vi "Robot Main.vi"() -> ()   [LabVIEW 2011]
doc: "This VI imlements the framework and scheduler for your robotics program. It should not be necessary to modify the framework. You are expected to add your code to the VIs called from Robot Main, the ones located in the Team Code within the project."
uses:
  <vilib>/Rock Robotics/WPI/Camera/WPI_CameraImageSize.ctl
  Robot Global Data.vi
panel:
  out "Timings":cluster{"Call Name":string, "Delta (ms)":u32}[](array[cluster])
  in  "Image Size":T1=enum."320x240"
  in  "Enable Vision":bool
  in  "Finish":bool
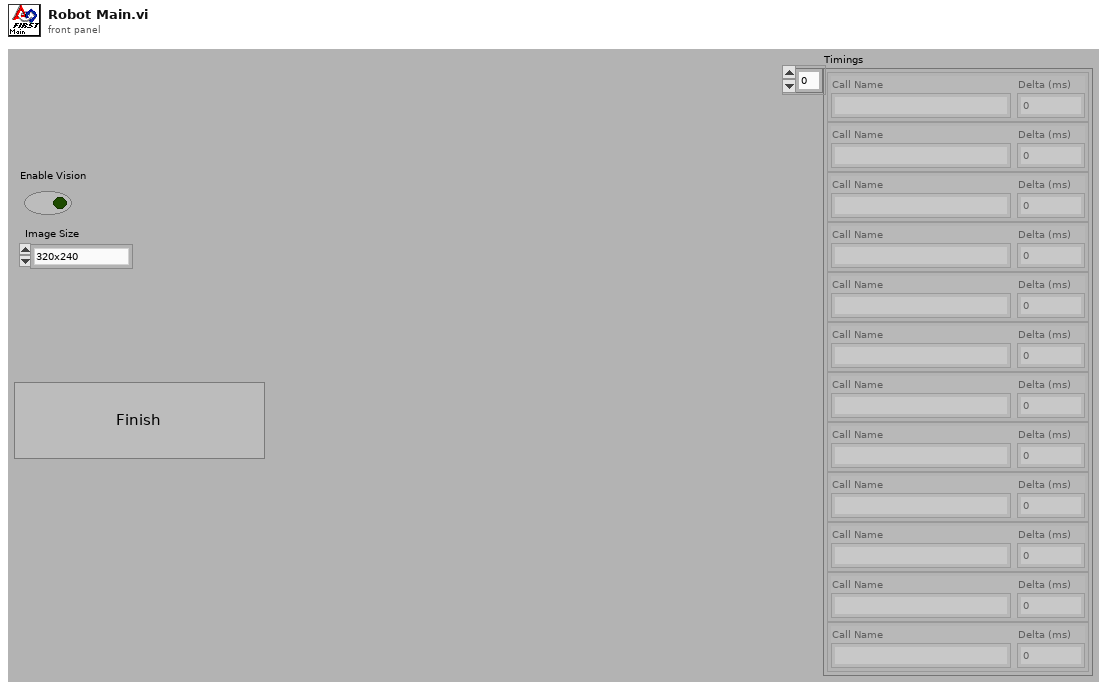
[diagram p1: front panel]
types:
  T1 = typedef "WPI_CameraImageSize.ctl" = enum16{"640x480", "320x240", "160x120"}
  T2 = typedef "WPI_DriverStationMatch Info.ctl" = cluster{"Autonomous Elapsed Seconds":dbl, "TeleOp Elapsed Seconds":dbl, "Disabled Elapsed Seconds":dbl, "Visited Autonomous":bool, "Visited TeleOp":bool, "Visited Disabled":bool, "Autonomous Settings":cluster{"Autonomous Style":enum16{"Iterative", "Independent"}, "VI Refnum":refnum<vi>}}
  T3 = typedef "WPI_DriverStationDerivedRobotMode.ctl" = enum16{"Init", "Execute", "Stop"}
  T4 = typedef "WPI_DriverStationRobotMode.ctl" = enum16{"Autonomous Disabled", "Autonomous Enabled", "Teleop Disabled", "Teleop Enabled", "Timeout", "Finish"}
  T5 = typedef "WPI_EncoderDevRef.ctl" = cluster{"DevStatus":errorcluster, "EncoderIndex":T6, "CounterIndex":T7, "DistancePerCount":dbl, "Decoding Type":T8}
  T6 = typedef "FPGA_EncoderIdx.ctl" = enum8{"Enc 0", "Enc 1", "Enc 2", "Enc 3", "Invalid"}
  T7 = typedef "FPGA_CounterCtrSystemIndex.ctl" = enum8{"Ctr 0", "Ctr 1", "Ctr 2", "Ctr 3", "Ctr 4", "Ctr 5", "Ctr 6", "Ctr 7", "Invalid"}
  T8 = typedef "WPI_EncoderType.ctl" = enum16{"1x", "2x", "4x"}
  T9 = typedef "WPI_GyroDevRef.ctl" = cluster{"DevStatus":errorcluster, "Analog Module":T10, "Analog Channel":T11, "Offset":dbl, "Gain (VoltsPerDegree/Second)":dbl}
  T10 = typedef "FPGA_TypedefAnalogModule.ctl" = enum16{"Analog Module 1", "Analog Module 2"}
  T11 = typedef "FPGA_AIChannel.ctl" = enum8{"AI 1", "AI 2", "AI 3", "AI 4", "AI 5", "AI 6", "AI 7", "AI 8", "Invalid"}
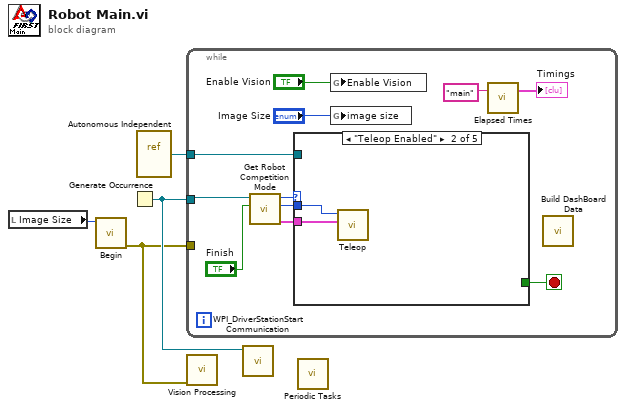
[diagram p0: block diagram]
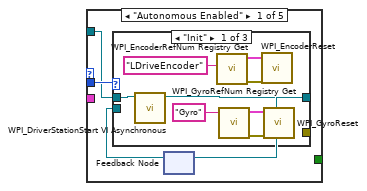
[diagram p2: hidden frame]
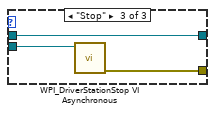
[diagram p4: hidden frame]
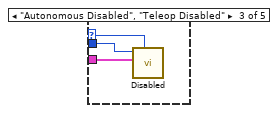
[diagram p5: hidden frame]
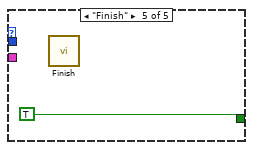
[diagram p7: hidden frame]
diagram:
  n1 = local read "Image Size"() -> (w3:T1)
  n2 = call "Begin.vi"("Image Size"=w3) -> ("error out"=w1:errorcluster)  [unwired: 10 out]
  n3 = Generate Occurrence() -> (w4:refnum<k4>)
  n4 = vi-ref "Autonomous Independent.vi"() -> (w2:refnum<vi>)
  n5 = while {
    tunnel: w4 -> [w13]
    tunnel: w1 -> [_]
    tunnel: w2 -> [w8]
    stop <- w10 stop-if-true
    n6 = call "Get Robot Competition Mode.vi"("Finish"="Finish", "DS Occurrence"=w13) -> ("Match Info out"=w11:T2, "Call Context"=w15:T3, "Robot Mode"=w14:T4)  [unwired: 7 out]
    n7 = case shown="\"Teleop Enabled\"" w14 {
      selector: w14 -> [_ _ w34 _ _]
      tunnel: w15 -> [w19 w33 w36 _ _]
      tunnel: w11 -> [_ w32 w35 _ _]
      tunnel: [_ _ _ _ TRUE] -> w10
      tunnel: w8 -> [w18 _ _ _ _]
      frame "Autonomous Enabled" {
        n8 = feedback #1() -> (w16:refnum<vi>)  [unwired: 1 out]
        n9 = case shown="\"Init\"" w19 {
          tunnel: w18 -> [w27 _ w30]
          tunnel: [w26 w28 w30] -> w17
          tunnel: w16 -> [_ w28 w31]
          tunnel: [_ _ w29] -> _
          frame "Init" {
            n10 = call <vilib>:"WPI_DriverStationStart VI Asynchronous.vi"("VI"=w27) -> ("VI out"=w26:refnum<vi>)  [unwired: 10 out]
            n11 = call <vilib>:"WPI_EncoderRefNum Registry Get.vi"("refnum name"="LDriveEncoder") -> ("error out"=w25:errorcluster, "EncoderDevRef"=w24:T5)  [unwired: 9 in]
            n12 = call <vilib>:"WPI_GyroRefNum Registry Get.vi"("refnum name"="Gyro") -> ("error out"=w22:errorcluster, "GyroDevRef"=w23:T9)  [unwired: 9 in]
            n13 = call <vilib>:"WPI_EncoderReset.vi"("error in (no error)"=w25, "EncoderDevRef"=w24) -> ()  [unwired: 8 in, 2 out]
            n14 = call <vilib>:"WPI_GyroReset.vi"("error in (no error)"=w22, "GyroDevRef"=w23) -> ()  [unwired: 8 in, 2 out]
          }
          frame "Execute", Default {
            # "Nothing to do"
          }
          frame "Stop" {
            n15 = call <vilib>:"WPI_DriverStationStop VI Asynchronous.vi"("VI Refnum"=w31) -> ("error out"=w29:errorcluster)  [unwired: 10 out]
          }
        }
        n16 = feedback-in #1(w17) -> ()
      }
      frame "Teleop Enabled" {
        n17 = call "Teleop.vi"("Match Info"=w32, "Call Context"=w33) -> ()  [unwired: 1 in, 9 out]
      }
      frame "Autonomous Disabled", "Teleop Disabled" {
        n18 = call "Disabled.vi"("Robot Mode"=w34, "Match Info"=w35, "Call Context"=w36) -> ()  [unwired: 1 in, 8 out]
      }
      frame "Timeout" {
      }
      frame "Finish" {
        n19 = call "Finish.vi"() -> ()  [unwired: 1 in, 7 out]
      }
    }
    n20 = global write "Robot Global Data.vi" "Enable Vision"("Enable Vision") -> ()
    n21 = global write "Robot Global Data.vi" "image size"("Image Size") -> ()
    n22 = call "Elapsed Times.vi"("Call Name"="main") -> ("Timings"=→"Timings":cluster{"Call Name":string, "Delta (ms)":u32}[])  [unwired: 2 in]
    n23 = call "Build DashBoard Data.vi"() -> ()  [unwired: 1 in, 11 out]
  }
  n24 = call "Vision Processing.vi"("error in (no error)"=w1) -> ()  [unwired: 1 in, 6 out]
  n25 = call <vilib>:"WPI_DriverStationStart Communication.vi"("occurrence"=w4) -> ()  [unwired: 11 out]
  n26 = call "Periodic Tasks.vi"() -> ()  [unwired: 2 in, 10 out]
